vi "Page_Exclusions_Initialize.vi"(8 "error in (no error)":errorcluster, 9 "ctlReferences":T1, 11 "AB_PackedLibrary in":refnum<class "AB_PackedLibrary.lvclass">) -> (0 "error out":errorcluster, 3 "AB_PackedLibrary out":refnum<class "AB_PackedLibrary.lvclass">)   [LabVIEW 2020, in "AB_PackedLibrary.lvclass"]
uses:
  <vilib>/AppBuilder/AB_Classes/PackedLib/AB_PackedLibrary.lvclass
  <resource>/Framework/Providers/Builds/AppBuilder/AB_UI_Page_Exclusions_References.ctl
  <vilib>/AppBuilder/AB_Classes/TargetFile/AB_Targetfile.lvclass
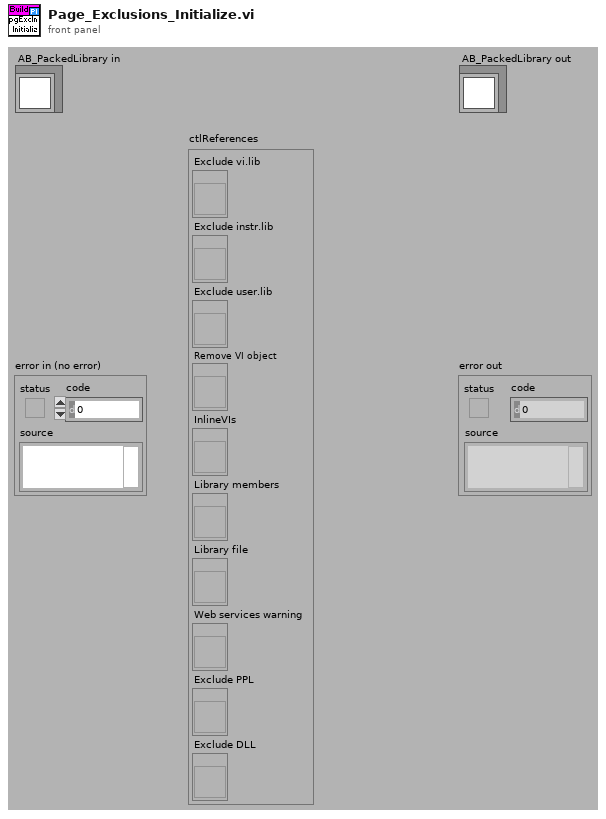
[diagram p1: front panel]
types:
  T1 = typedef "AB_UI_Page_Exclusions_References.ctl" = cluster{"Exclude vi.lib":refnum<vi>, "Exclude instr.lib":refnum<vi>, "Exclude user.lib":refnum<vi>, "Remove VI object":refnum<vi>, "InlineVIs":refnum<vi>, "Library members":refnum<vi>, "Library file":refnum<vi>, "Web services warning":refnum<vi>, "Exclude PPL":refnum<vi>, "Exclude DLL":refnum<vi>}
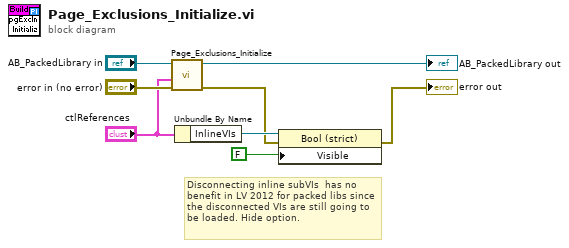
[diagram p0: block diagram]
diagram:
  # "Disconnecting inline subVIs  has no benefit in LV 2012 for packed libs since the disconnected VIs are still going to be loaded. Hide option."
  n1 = call-parent "Page_Exclusions_Initialize.vi"("error in (no error)"="error in (no error)", "ctlReferences"="ctlReferences", "AB_Targetfile in"="AB_PackedLibrary in") -> ("error out"=w2:errorcluster, "AB_Targetfile out"=→"AB_PackedLibrary out":refnum<class "AB_PackedLibrary.lvclass">)  [unwired: 7 in]
  n2 = Unbundle By Name("ctlReferences") -> ("InlineVIs"=w3:refnum<vi>)
  n3 = property class="Bool (strict)"(reference=w3, error in=w2, "Visible"=FALSE) -> (error out=→"error out":errorcluster)  [unwired: 1 out]
